vi "DecodeMaskedBytes.vi"(8 "error in (no error)":errorcluster, 10 "Mask Bytes":string, 11 "Encoded Data":string) -> (0 "error out":errorcluster, 3 "Decoded Data":string)   [LabVIEW 2014, in "QwaveSys RPi Training Library.lvlib" / "WebSockets.lvlib"]
doc: "Unmasks incoming data. Data sent to the client does not need to be masked.\nWebSockets API 1.3.0.13\nSam Sharp - Intelligent Energy\nCopyright (c) 2015, Intelligent Energy"
uses:
  <vilib>/Q-Wave Systems/QwaveSys RPi Training Package (Demo)/Addons/WebSockets API/WebSockets/WebSockets.lvlib
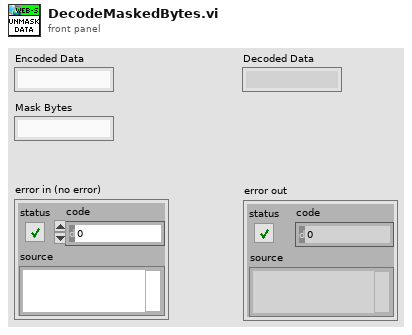
[diagram p1: front panel]
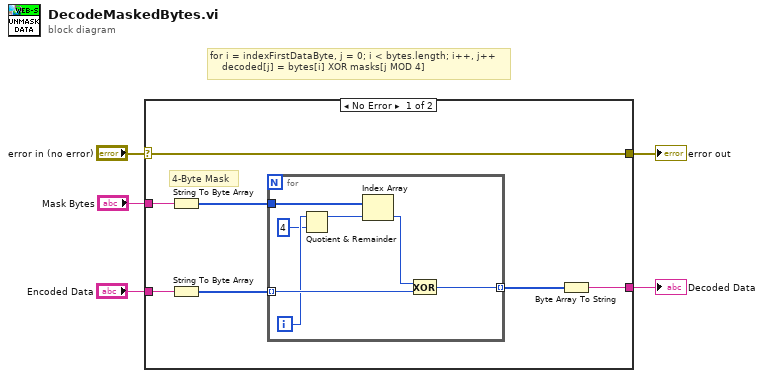
[diagram p0: block diagram]
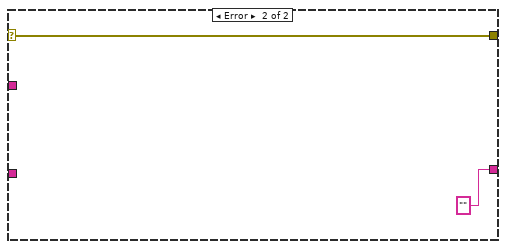
[diagram p2: hidden frame]
diagram:
  # "for i = indexFirstDataByte, j = 0; i < bytes.length; i++, j++\n    decoded[j] = bytes[i] XOR masks[j MOD 4]"
  n1 = case shown="No Error" "error in (no error)" {
    selector: "error in (no error)" -> [w12 w21]
    tunnel: "Encoded Data" -> [w10 _]
    tunnel: "Mask Bytes" -> [w11 _]
    tunnel: [w9 "" ("Mask Bytes")] -> w5
    tunnel: [w12 w21] -> w1
    frame No Error {
      # "4-Byte Mask"
      n2 = String To Byte Array(string=w11) -> (unsigned byte array=w7:u8[])
      n3 = String To Byte Array(string=w10) -> (unsigned byte array=w8:u8[])
      n4 = for {
        tunnel: w8 -> [w19] mode=indexing
        tunnel: w7 -> [w15]
        tunnel: [w13] -> w6 mode=indexing
        i -> [w18]
        n5 = Quotient & Remainder(x=w18, y=4) -> (x-y*floor(x/y)=w16:i32)  [unwired: 1 out]
        n6 = Index Array(array=w15, index=w16) -> (element=w14:u8)
        n7 = Exclusive Or(1:w19, 2:w14) -> (0:w13:u8)
      }
      n8 = Byte Array To String(unsigned byte array=w6) -> (string=w9:string)
    }
    frame Error {
    }
  }
  "Decoded Data" <- w5
  "error out" <- w1
